vi "Error Process.vi"(8 "error in (no error)":errorcluster, 11 "Variables":T1) -> (0 "error out":errorcluster)   [LabVIEW 2017]
uses:
  support/Controls/Shared Variables.ctl
  Configuration/Controls/ConfigData.ctl
  Elevator/Controls/Elevator Overhead.ctl
  Elevator/Controls/Elevator States.ctl
  Elevator/Controls/Elevator Location.ctl
  Elevator/Controls/Elevator Command Event.ctl
  Elevator/Controls/Elevator Commands.ctl
  Controls/Error EventData.ctl
  Controls/Error Type.ctl
  support/Controls/User Events.ctl
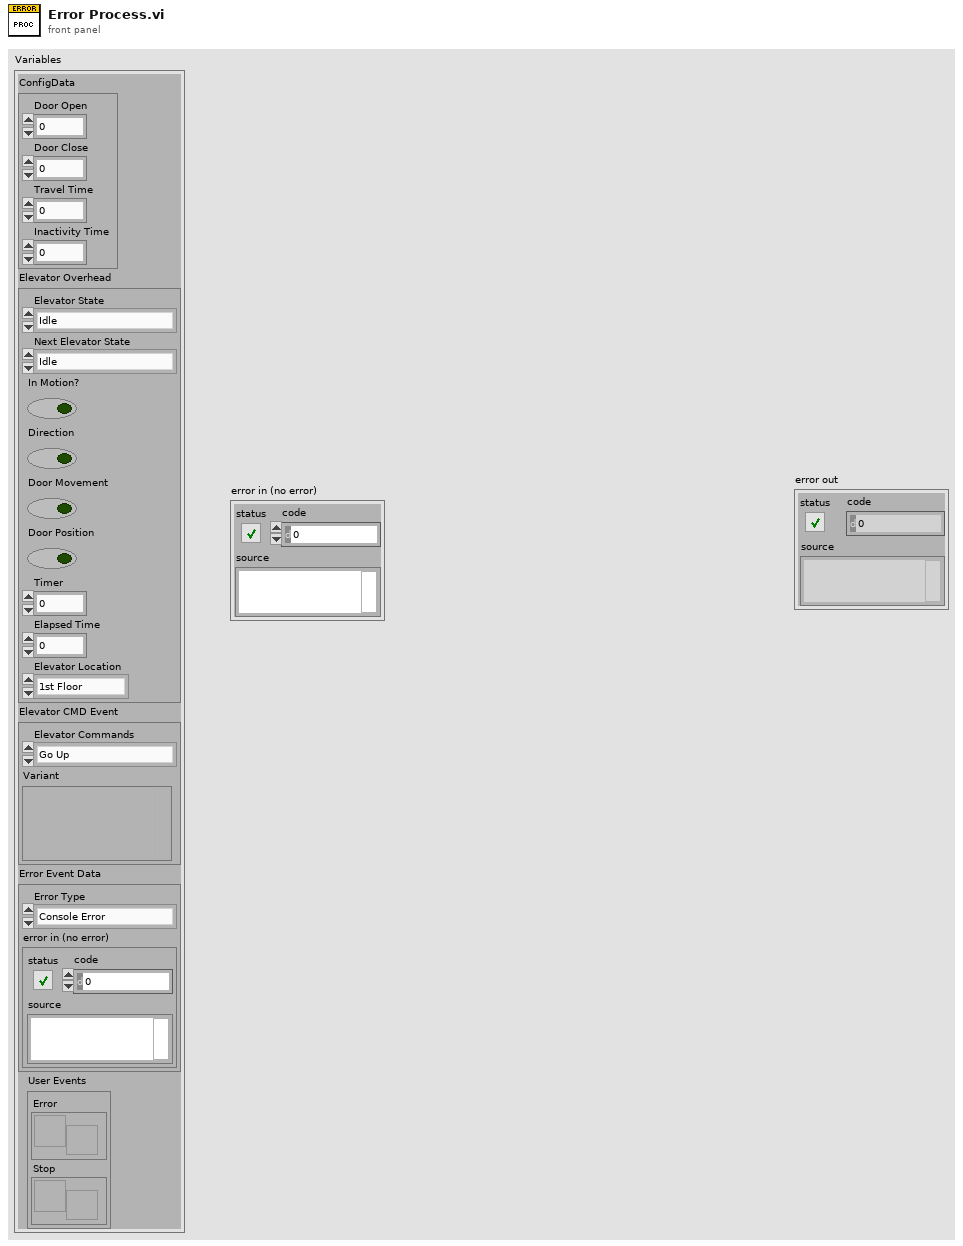
[diagram p1: front panel]
types:
  T1 = typedef "Shared Variables.ctl" = cluster{"ConfigData":T2, "Elevator Overhead":T3, "Elevator CMD Event":T6, "Error Event Data":T8, "User Events":T10}
  T2 = typedef "ConfigData.ctl" = cluster{"Door Open":dbl, "Door Close":dbl, "Travel Time":dbl, "Inactivity Time":dbl}
  T3 = typedef "Elevator Overhead.ctl" = cluster{"Elevator State":T4, "Next Elevator State":T4, "In Motion?":bool, "Direction":bool, "Door Movement":bool, "Door Position":bool, "Timer":dbl, "Elapsed Time":dbl, "Elevator Location":T5}
  T4 = typedef "Elevator States.ctl" = enum16{"Idle", "Init", "Open Doors", "Close Doors", "Start Move", "Move", "Finish Move", "Analysis", "Emergency"}
  T5 = typedef "Elevator Location.ctl" = enum16{"1st Floor", "2nd Floor", "3rd Floor", "4th Floor"}
  T6 = typedef "Elevator Command Event.ctl" = cluster{"Elevator Commands":T7, "Variant":variant}
  T7 = typedef "Elevator Commands.ctl" = enum16{"Go Up", "Go Down", "Go to Floor", "Emergency", "Open Doors", "Close Doors"}
  T8 = typedef "Error EventData.ctl" = cluster{"Error Type":T9, "error in (no error)":errorcluster}
  T9 = typedef "Error Type.ctl" = enum16{"Console Error", "Sensor Interface IO Error", "Process Step Error"}
  T10 = typedef "User Events.ctl" = cluster{"Error":refnum<user-event>, "Stop":refnum<user-event>}
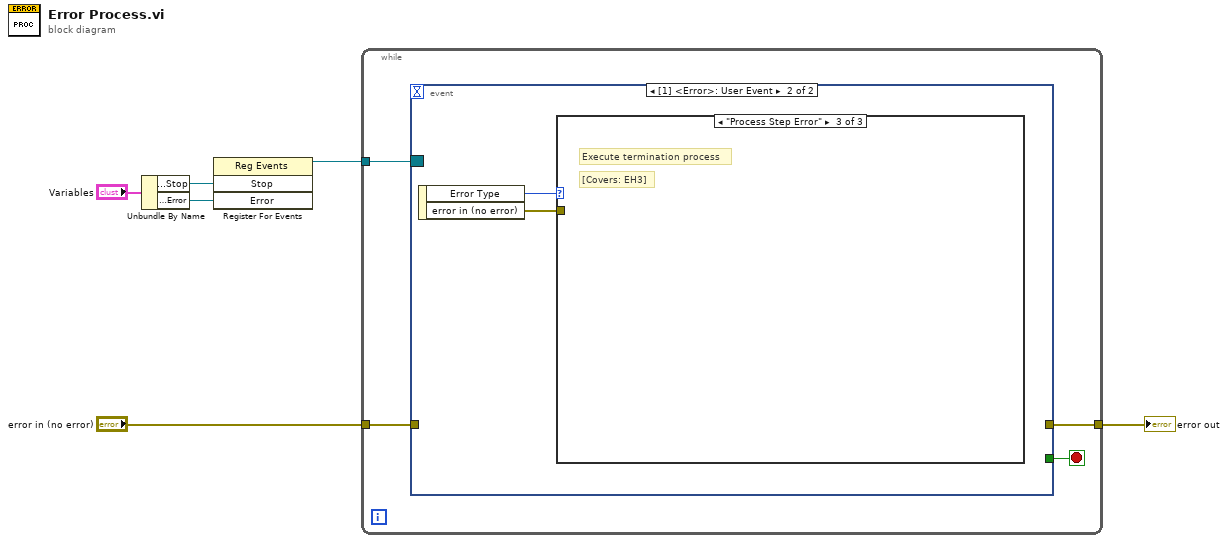
[diagram p0: block diagram]
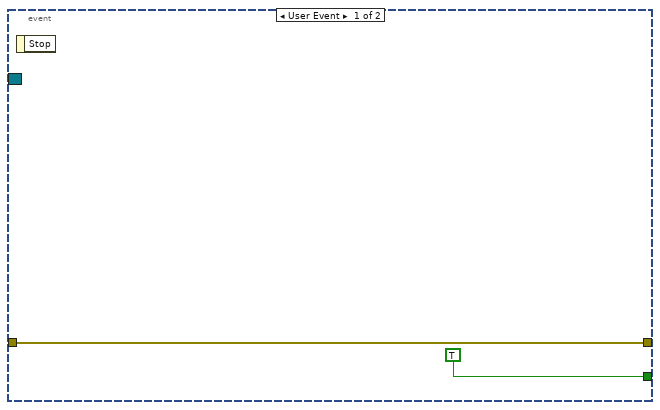
[diagram p2: hidden frame]
diagram:
  n1 = Unbundle By Name("Variables") -> ("User Events.Stop"=w5:refnum<user-event>, "User Events.Error"=w1:refnum<user-event>)
  n2 = register-events(w5, w1) -> (reference out=w4:refnum<event-registration>)  [unwired: 2 in, 1 out]
  n3 = while {
    tunnel: w4 -> [w10]
    tunnel: "error in (no error)" -> [w8]
    tunnel: [w7] -> w3
    stop <- w9 stop-if-true
    n4 = event shown="[1] <Error>: User Event" {
      selector: w10 -> [_ _]
      dyn-events: _ -> [_ _]
      timeout: _ -> [_ _]
      tunnel: [TRUE _] -> w9
      tunnel: w8 -> [w11 _]
      tunnel: [w11 _] -> w7
      event User Event {
        n5 = event-data() -> ()  [unwired: 1 in, 1 out]
      }
      event User Event {
        n6 = event-data() -> ("Error Type"=w14:T9, "error in (no error)"=w13:errorcluster)  [unwired: 1 in]
        n7 = case shown="\"Process Step Error\"" w14 {
          tunnel: w13 -> [_ _ _]
          frame "Console Error", Default {
            # "[Covers: EH1B2]"
            # "If continue, process error as a \"Process Step Error\""
            # "[Covers: EH1B1]"
            # "If error cleared, continue last operation"
            # "[Covers: EH1B]"
            # "If error source = User Console, allow user to choose to clear or continue w/error"
            # "[Covers: EH1A]"
            # "If error source = Display Console, notify user and clear error"
            # "[Covers: EH1]"
            # "Console Error = Alert user without interuption of elevator"
          }
          frame "Sensor Interface IO Error" {
            # "[Covers: EH2]"
            # "Execute termination process"
          }
          frame "Process Step Error" {
            # "[Covers: EH3]"
            # "Execute termination process"
          }
        }
      }
    }
  }
  "error out" <- w3
